vi "ex_tdsReadAllProperties.vi"(4 "error in (no error)":errorcluster, 7 "Data Object in":refnum<k20>) -> (0 "error out":errorcluster, 1 "Properties Out":T2[](array[typedef]), 3 "Data Object out":refnum<k20>)   [LabVIEW 2020]
uses:
  <vilib>/express/express shared/ExFile.llb/ex_TdmProperty.ctl
  <vilib>/express/express shared/ex_EditUserDefinedProperties/usiDataType.ctl
  <vilib>/Platform/storage/lvStorage.llb/_internalProps.ctl
  <vilib>/Platform/storage/Storage.llb/__loadPropRefList.vi
  <vilib>/Platform/storage/Storage.llb/Get Property (I32).vi
  <vilib>/Platform/storage/Storage.llb/Get Property (DBL).vi
  <vilib>/Platform/storage/Storage.llb/Get Property (Time Stamp).vi
  <vilib>/Platform/storage/Storage.llb/Get Property (String).vi
  <vilib>/Platform/storage/Storage.llb/Get Property (Enum).vi
  <vilib>/Platform/storage/Storage.llb/__loadPropString.vi
  <vilib>/Platform/storage/Storage.llb/__loadPropFloat64.vi
  <vilib>/Platform/storage/Storage.llb/__loadPropInt32.vi
  <vilib>/Platform/storage/Storage.llb/__loadPropTime.vi
  <resource>/objmgr/Storage.rc
panel:
  in  "DNL_Property names":T1=["wf_start_time", "wf_increment", "wf_xname", "wf_xunit_string", "wf_start_offset", "wf_time_pref", "wf_samples", "wf_create_time", "wf_xcolumns"]
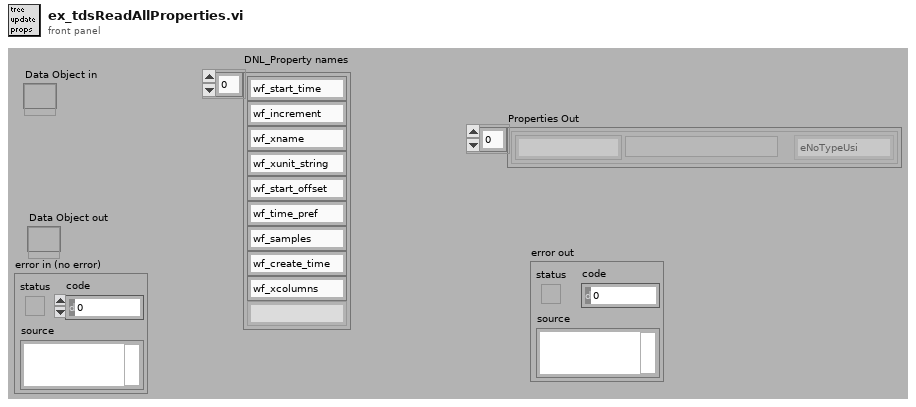
[diagram p1: front panel]
types:
  T1 = typedef "_internalProps.ctl" = string[]
  T2 = typedef "ex_TdmProperty.ctl" = cluster{"Name":string, "Type":T3, "Value":variant}
  T3 = typedef "usiDataType.ctl" = enum16{"eNoTypeUsi", "eInt8Usi", "eInt16Usi", "eInt32Usi", "eInt64Usi", "eUInt8Usi", "eUInt16Usi", "eUInt32Usi", "eUInt64Usi", "eFloat32Usi", "eFloat64Usi", "- 0", "- 1", "- 2", "- 3", "- 4", "- 5", "- 6", "- 7", "- 8", "- 9", "eString8Usi", "eString16Usi", "eStringUsi", "eEnumUsi", "- 10", "- 11", "- 12", "- 13", "- 14", "eTimeUsi", "- 15", "- 16", "- 17", "- 18", "- 19", "- 20", "- 21", "- 22", "- 23", "eInstanceUsi", "eStoreUsi"}
  T4 = typedef "usiPropDef.ctl" = cluster{"name":string, "baseName":string, "refDataType":string, "dimensions":i32, "type":i32, "user defined":bool, "enumStrings":string[], "usiDataType":T3, "specialProp":T5, "Property Source":string, "index":i32}
  T5 = typedef "specialProperties.ctl" = enum16{"<Default>", "Channel Values", "AppendReplace", "ChannelFlags", "ValueFlags", "ImplicitExplicit", "InsertIndex", "ValuesCount", "ComparisonOperator", "Cluster", "DAQmx Channel"}
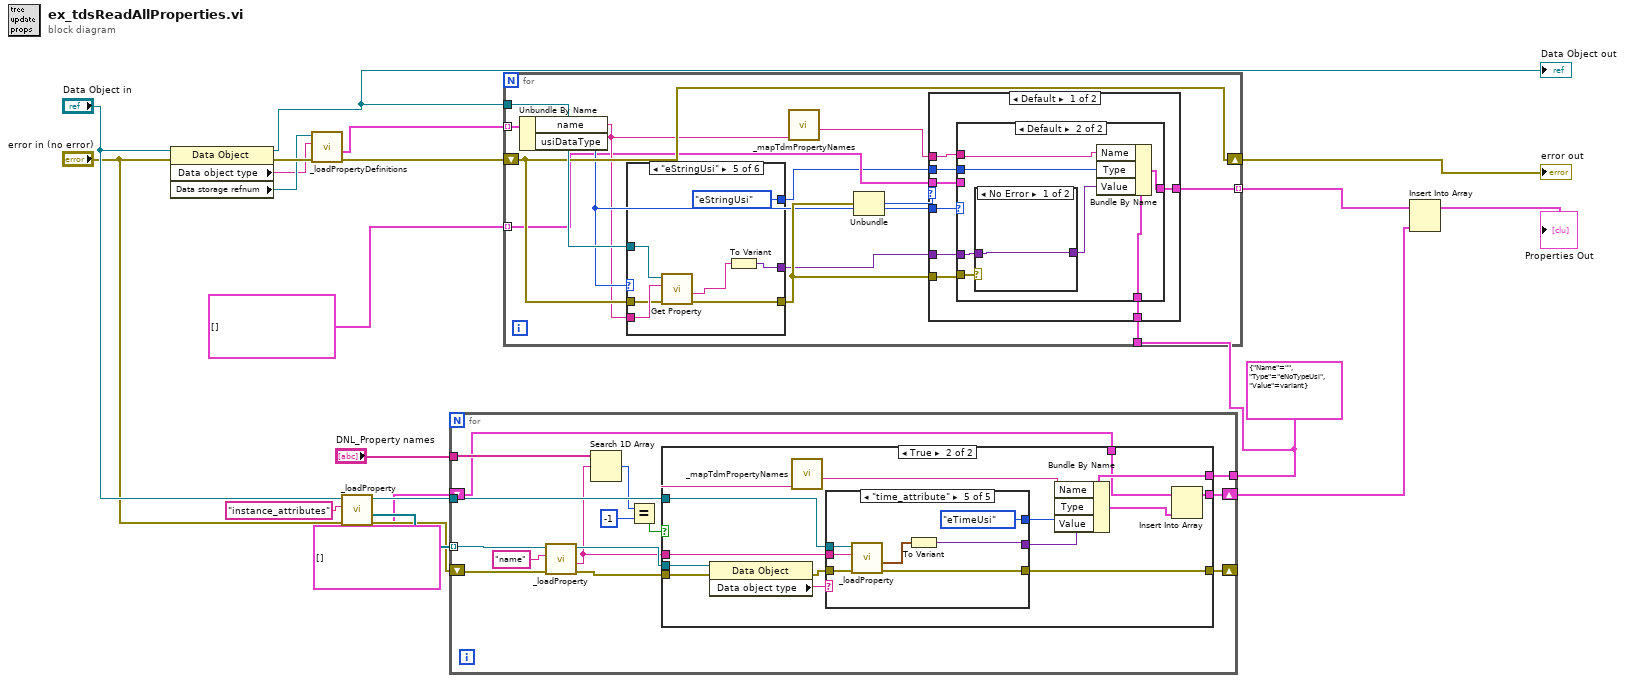
[diagram p0: block diagram]
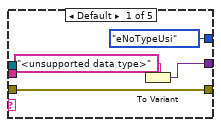
[diagram p3: hidden frame]
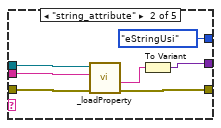
[diagram p4: hidden frame]
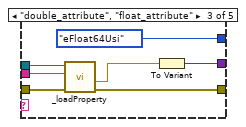
[diagram p5: hidden frame]
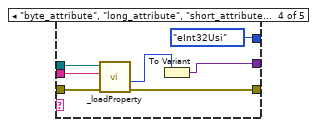
[diagram p6: hidden frame]
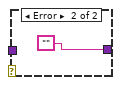
[diagram p8: hidden frame]
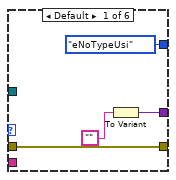
[diagram p10: hidden frame]
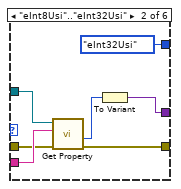
[diagram p11: hidden frame]
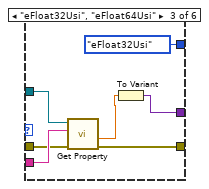
[diagram p12: hidden frame]
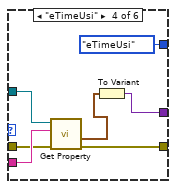
[diagram p13: hidden frame]
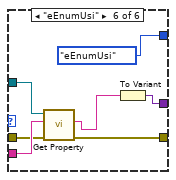
[diagram p14: hidden frame]
diagram:
  w5 = T2 {"Name"="", "Type"=enum."eNoTypeUsi", "Value"=variant} ("TDM Property")
  n1 = property class="Data Object"(reference="Data Object in", error in="error in (no error)") -> (reference out=w16:refnum<k20>, error out=w19:errorcluster, "Data object type"=w17:string, "Data storage refnum"=w18:refnum<k20>)
  "Data Object out" <- w16
  n2 = call <vilib>:"_loadPropertyDefinitions.vi"("error in (no error)"=w19, "Object type"=w17, "storage refnum"=w18) -> ("error out"=w15:errorcluster, "PropertyDefinitions"=w14:T4[])  [unwired: 1 in, 2 out]
  n3 = call-poly <vilib>:"_loadProperty.vi"("error in (no error)"="error in (no error)", "Property name"="instance_attributes" ("PropertyName"), "storage refnum"="Data Object in") -> ("error out"=w11:errorcluster, "Value"=w12:refnum<k20>[], "dup storage refnum"=w10:refnum<k20>)  [unwired: 6 out]
  n4 = for {
    tunnel: w12 -> [w35] mode=indexing
    shift-right: [w32] -> _
    shift-left: w11 -> [w33]
    tunnel: w10 -> [w31]
    tunnel: w5 -> [w28]
    tunnel: "DNL_Property names" -> [w27]
    shift-right: [w25] -> w3
    shift-left: T2[] [] -> [w24]
    n5 = call-poly <vilib>:"_loadProperty.vi"("error in (no error)"=w33, "Property name"="name", "storage refnum"=w35) -> ("error out"=w29:errorcluster, "Value"=w26:string, "dup storage refnum"=w30:refnum<k20>)  [unwired: 6 out]
    n6 = Search 1D Array(1D array=w27, element=w26) -> (index of element=w23:i32)  [unwired: 1 out]
    n7 = Equal?(x=w23, y=-1) -> (x = y?=w21:bool)
    n8 = case shown="True" w21 {
      tunnel: [w36 w51] -> w32
      tunnel: w31 -> [_ w50]
      tunnel: w30 -> [_ w49]
      tunnel: w29 -> [w36 w48]
      tunnel: w28 -> [_ w42]
      tunnel: w26 -> [_ w41]
      tunnel: [w37 w39] -> w25
      tunnel: w24 -> [w37 w38]
      frame False {
      }
      frame True {
        n9 = property class="Data Object"(reference=w49, error in=w48) -> (error out=w46:errorcluster, "Data object type"=w47:string)  [unwired: 1 out]
        n10 = call <vilib>:"_mapTdmPropertyNames.vi"("DNL_Name_in"=w41) -> ("DNL_Mapped_Name_out"=w45:string)  [unwired: 3 in, 3 out]
        n11 = case shown="\"time_attribute\"" w47 {
          tunnel: [w55 w62 w69 w76 w83] -> w51
          tunnel: w50 -> [_ w61 w68 w75 w82]
          tunnel: w41 -> [_ w60 w67 w74 w81]
          tunnel: w46 -> [w55 w59 w66 w73 w80]
          tunnel: [usiDataType."eNoTypeUsi" ("Type") usiDataType."eStringUsi" ("Type") usiDataType."eFloat64Usi" ("Type") usiDataType."eInt32Usi" ("Type") usiDataType."eTimeUsi" ("Type")] -> w44
          tunnel: [w52 w56 w63 w70 w77] -> w43
          frame Default {
            n12 = To Variant(anything="<unsupported data type>" ("Value")) -> (Variant=w52:variant)
          }
          frame "string_attribute" {
            n13 = call-poly <vilib>:"_loadProperty.vi"("error in (no error)"=w59, "Property name"=w60, "storage refnum"=w61) -> ("error out"=w62:errorcluster, "Value"=w57:string)  [unwired: 7 out]
            n14 = To Variant(anything=w57) -> (Variant=w56:variant)
          }
          frame "double_attribute", "float_attribute" {
            n15 = call-poly <vilib>:"_loadProperty.vi"("error in (no error)"=w66, "Property name"=w67, "storage refnum"=w68) -> ("error out"=w69:errorcluster, "Value"=w64:dbl)  [unwired: 7 out]
            n16 = To Variant(anything=w64) -> (Variant=w63:variant)
          }
          frame "byte_attribute", "long_attribute", "short_attribute" {
            n17 = call-poly <vilib>:"_loadProperty.vi"("error in (no error)"=w73, "Property name"=w74, "storage refnum"=w75) -> ("error out"=w76:errorcluster, "Value"=w71:i32)  [unwired: 7 out]
            n18 = To Variant(anything=w71) -> (Variant=w70:variant)
          }
          frame "time_attribute" {
            n19 = call-poly <vilib>:"_loadProperty.vi"("error in (no error)"=w80, "Property name"=w81, "storage refnum"=w82) -> ("error out"=w83:errorcluster, "Value"=w78:timestamp)  [unwired: 7 out]
            n20 = To Variant(anything=w78) -> (Variant=w77:variant)
          }
        }
        n21 = Bundle By Name(cluster=w42, "Name"=w45, "Type"=w44, "Value"=w43) -> (w40:T2)
        n22 = Insert Into Array(array=w38, new element=w40) -> (w39:T2[])  [unwired: 1 in]
      }
    }
  }
  n23 = for {
    shift-right: [w92] -> w20
    shift-left: w15 -> [w92]
    tunnel: w16 -> [w96]
    tunnel: w14 -> [w93] mode=indexing
    tunnel: T2[] [] -> [w85] mode=indexing
    tunnel: w5 -> [w88]
    tunnel: [w87] -> w4 mode=indexing
    n24 = Unbundle By Name(w93) -> ("name"=w90:string, "usiDataType"=w91:T3)
    n25 = case shown="\"eStringUsi\"" w91 {
      tunnel: w90 -> [_ w126 w133 w140 w147 w154]
      tunnel: w92 -> [w119 w125 w132 w139 w146 w153]
      tunnel: [w119 w124 w131 w138 w145 w152] -> w95
      tunnel: w96 -> [_ w123 w130 w137 w144 w151]
      tunnel: [w117 w121 w128 w135 w142 w149] -> w86
      tunnel: [usiDataType."eNoTypeUsi" ("Type") usiDataType."eInt32Usi" ("Type") usiDataType."eFloat32Usi" ("Type") usiDataType."eTimeUsi" ("Type") usiDataType."eStringUsi" ("Type") usiDataType."eEnumUsi" ("Type")] -> w84
      frame Default {
        n26 = To Variant(anything="") -> (Variant=w117:variant)
      }
      frame "eInt8Usi".."eInt32Usi" {
        n27 = call-poly <vilib>:"Get Property.vi"("error in (no error)"=w125, "Property name"=w126, "storage refnum"=w123) -> ("error out"=w124:errorcluster, "Value"=w122:i32)  [unwired: 7 out]
        n28 = To Variant(anything=w122) -> (Variant=w121:variant)
      }
      frame "eFloat32Usi", "eFloat64Usi" {
        n29 = call-poly <vilib>:"Get Property.vi"("error in (no error)"=w132, "Property name"=w133, "storage refnum"=w130) -> ("error out"=w131:errorcluster, "Value"=w129:dbl)  [unwired: 7 out]
        n30 = To Variant(anything=w129) -> (Variant=w128:variant)
      }
      frame "eTimeUsi" {
        n31 = call-poly <vilib>:"Get Property.vi"("error in (no error)"=w139, "Property name"=w140, "storage refnum"=w137) -> ("error out"=w138:errorcluster, "Value"=w136:timestamp)  [unwired: 7 out]
        n32 = To Variant(anything=w136) -> (Variant=w135:variant)
      }
      frame "eStringUsi" {
        n33 = call-poly <vilib>:"Get Property.vi"("error in (no error)"=w146, "Property name"=w147, "storage refnum"=w144) -> ("error out"=w145:errorcluster, "Value"=w143:string)  [unwired: 7 out]
        n34 = To Variant(anything=w143) -> (Variant=w142:variant)
      }
      frame "eEnumUsi" {
        n35 = call-poly <vilib>:"Get Property.vi"("error in (no error)"=w153, "Property name"=w154, "storage refnum"=w151) -> ("error out"=w152:errorcluster, "String"=w150:string)  [unwired: 7 out]
        n36 = To Variant(anything=w150) -> (Variant=w149:variant)
      }
    }
    n37 = call <vilib>:"_mapTdmPropertyNames.vi"("DNL_Name_in"=w90) -> ("DNL_Mapped_Name_out"=w89:string)  [unwired: 3 in, 3 out]
    n38 = Unbundle(w95) -> ("code"=w94:i32)  [unwired: 2 out]
    n39 = case shown="Default" w94 {
      tunnel: w89 -> [w104 _]
      tunnel: w86 -> [w103 _]
      tunnel: w91 -> [w102 _]
      tunnel: w95 -> [w101 _]
      tunnel: w88 -> [w100 _]
      tunnel: [w99 w115] -> w87
      tunnel: w85 -> [w98 w115]
      tunnel: w84 -> [w97 _]
      frame Default {
        n40 = case shown="Default" w102 {
          tunnel: w104 -> [_ w109]
          tunnel: w103 -> [_ w111]
          tunnel: w101 -> [_ w112]
          tunnel: w100 -> [_ w108]
          tunnel: [w105 w107] -> w99
          tunnel: w98 -> [w105 _]
          tunnel: w97 -> [_ w106]
          frame "eInstanceUsi", "eStoreUsi" {
          }
          frame Default {
            n41 = case shown="No Error" w112 {
              tunnel: [w113 ""] -> w110
              tunnel: w111 -> [w113 _]
              frame No Error {
              }
              frame Error {
              }
            }
            n42 = Bundle By Name(cluster=w108, "Name"=w109, "Type"=w106, "Value"=w110) -> (w107:T2)
          }
        }
      }
      frame 2552 {
      }
    }
  }
  "error out" <- w20
  n43 = Insert Into Array(array=w4, new element=w3) -> (→"Properties Out":T2[])  [unwired: 1 in]
